vi "Global Y Border.vi"() -> ()   [LabVIEW 2014]
panel:
  out "GlobalYBorder":dbl=5.0
  # "GlobalYBorder is the amount of extra space on the field compared to ACTUAL \nfield as Intensity Graph. So if Global FieldWidthY = 50, then the  top rightmost corner is\nat y-coordinate 55 if GlobalXBorder is 5"
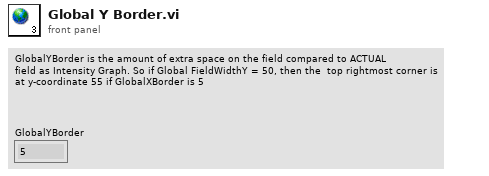
[diagram p1: front panel]
diagram:
